vi "GVHorstSP.vi"() -> ()   [LabVIEW 2010]
panel:
  out "HorstSP":dbl[](array[numeric])
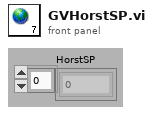
[diagram p1: front panel]
diagram:
